vi "FilterArray_Graphic_CH1_LP.vi"(4 "Window Size":dbl, 7 "Instantaneous BER":dbl) -> (0 "Slide Bar":dbl, 3 "Graph Instantaneous BER":dbl)   [LabVIEW 2022 SP3]
uses:
  <vilib>/Analysis/baseanly.llb/Mean (DBL).vi
  <vilib>/Analysis/NI_AALBase.lvlib
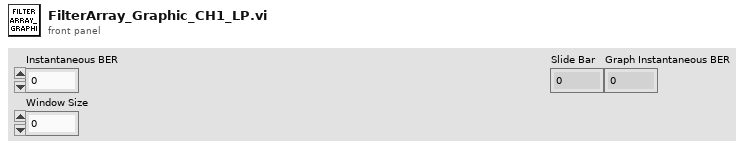
[diagram p1: front panel]
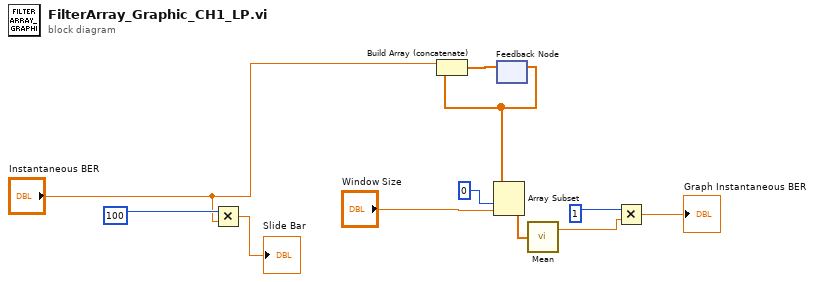
[diagram p0: block diagram]
diagram:
  n1 = Multiply(x=100, y="Instantaneous BER") -> (x*y=→"Slide Bar":dbl)
  n2 = feedback #1() -> (w4:dbl[])  [unwired: 1 in]
  n3 = Build Array (concatenate)("Instantaneous BER", w4) -> (w10:dbl[])
  n4 = Array Subset(array=w4, index=0, length="Window Size") -> (w9:dbl[])
  n5 = feedback-in #1(w10) -> ()
  n6 = call-poly <vilib>:"Mean.vi"("X"=w9) -> ("mean"=w2:dbl)  [unwired: 1 out]
  n7 = Multiply(x=1, y=w2) -> (x*y=→"Graph Instantaneous BER":dbl)
